vi "Stop.vi"(8 "error in (no error)":errorcluster, 11 "reference in":refnum<class "sim_MmW.lvclass">) -> (0 "error out":errorcluster, 3 "reference out":refnum<class "sim_MmW.lvclass">)   [LabVIEW 2019, in "sim_MmW.lvclass"]
doc: "Stop operation"
uses:
  sim_MmW.lvclass
  C:/Barkhausen mmWave radar/Development/LV/Barkhausen mmWave hardware control/Host/SubVIs/mmWave instrument_class/mmWave instrument.lvclass
  mmWave instrument_class/Instrument state.ctl
  mmWave instrument_class/mmWave instrument.lvclass
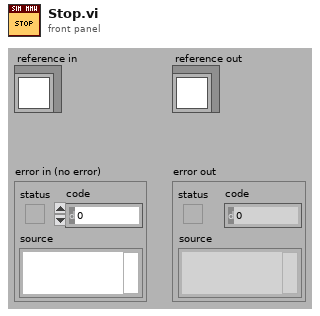
[diagram p1: front panel]
types:
  T1 = typedef "mmWave instrument.lvclass/Instrument state.ctl" = enum16{"Off", "Initialization", "Configuration", "Running", "Calibration"}
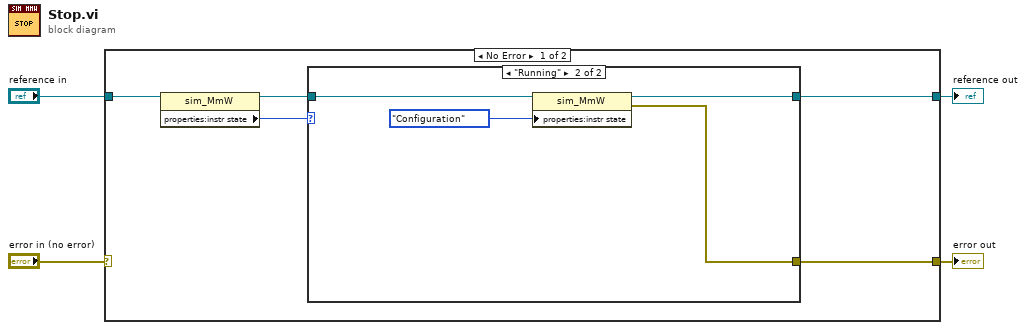
[diagram p0: block diagram]
diagram:
  n1 = case shown="No Error" "error in (no error)" {
    selector: "error in (no error)" -> [_ w16]
    tunnel: [w7 w16] -> w3
    tunnel: [w8 w15] -> w1
    tunnel: "reference in" -> [w9 w15]
    frame No Error {
      n2 = property class="sim_MmW"(reference=w9) -> (reference out=w6:refnum<class "sim_MmW.lvclass">, "properties:instr state"=w5:T1)  [unwired: 1 in, 1 out]
      n3 = case shown="\"Running\"" w5 {
        tunnel: [w10 w13] -> w8
        tunnel: [_ w11] -> w7
        tunnel: w6 -> [w10 w14]
        frame "Off", Default {
        }
        frame "Running" {
          n4 = property class="sim_MmW"(reference=w14, "properties:instr state"=Instrument_state."Configuration" ("instr state")) -> (reference out=w13:refnum<class "sim_MmW.lvclass">, error out=w11:errorcluster)  [unwired: 1 in]
        }
      }
    }
    frame Error {
    }
  }
  "error out" <- w3
  "reference out" <- w1
